vi "FrameTime.vi"(0 "Is Extended ID?":bool, 7 "DataLength":u32) -> ()   [LabVIEW 2014, in "CAN Bus Monitor Engine.lvlib"]
uses:
  BM Global Vars.vi
  CAN Bus Monitor Engine.lvlib
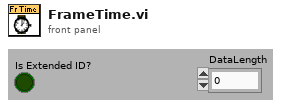
[diagram p1: front panel]
types:
  T1 = cluster{"IncMinFrameTime":dbl, "IncMaxFrameTime":dbl, "Min Frame Length":dbl[][], "Max Frame Length":dbl[][], "Std Frames":u32, "Ext Frames":u32, "Error Frames":u32, "Remote Frames":u32, "Std Frames / Sec":u32, "Ext Frames / Sec":u32, "Error Frames / Sec":u32, "Remote Frames / Sec":u32, "Peak Bus Load":dbl, "Bus Load":dbl, "Start Timestamp":dbl, "Null Frames":u32, "Null Frames / Sec":u32}
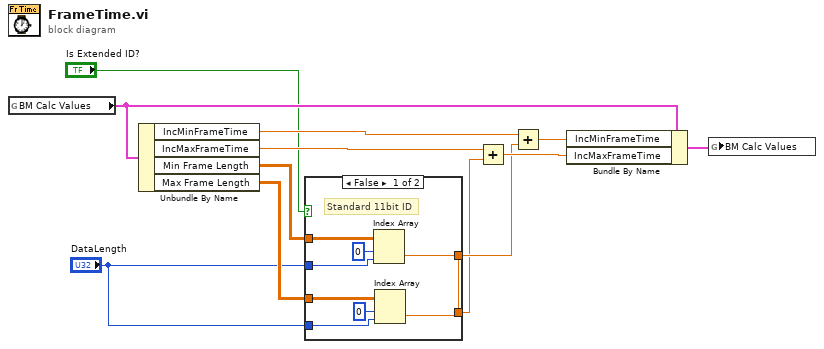
[diagram p0: block diagram]
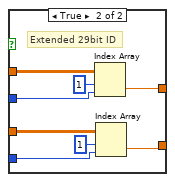
[diagram p2: hidden frame]
diagram:
  n1 = global read "BM Global Vars.vi" "BM Calc Values"() -> (w3:T1)
  n2 = Unbundle By Name(w3) -> ("IncMinFrameTime"=w12:dbl, "IncMaxFrameTime"=w11:dbl, "Min Frame Length"=w8:dbl[][], "Max Frame Length"=w7:dbl[][])
  n3 = case shown="False" "Is Extended ID?" {
    tunnel: "DataLength" -> [w18 w26]
    tunnel: "DataLength" -> [w17 w25]
    tunnel: [w16 w24] -> w4
    tunnel: [w15 w23] -> w5
    tunnel: w8 -> [w14 w22]
    tunnel: w7 -> [w13 w21]
    frame False {
      # "Standard 11bit ID"
      n4 = Index Array(array=w14, index (row)=0, index (col)=w18) -> (element=w16:dbl)
      n5 = Index Array(array=w13, index (row)=0, index (col)=w17) -> (element=w15:dbl)
    }
    frame True {
      # "Extended 29bit ID"
      n6 = Index Array(array=w22, index (row)=1, index (col)=w26) -> (element=w23:dbl)
      n7 = Index Array(array=w21, index (row)=1, index (col)=w25) -> (element=w24:dbl)
    }
  }
  n8 = Add(x=w11, y=w4) -> (x+y=w9:dbl)
  n9 = Add(x=w12, y=w5) -> (x+y=w10:dbl)
  n10 = Bundle By Name(cluster=w3, "IncMinFrameTime"=w10, "IncMaxFrameTime"=w9) -> (w2:T1)
  n11 = global write "BM Global Vars.vi" "BM Calc Values"(w2) -> ()
